vi "2014 Ball Detection.vi"(0 "Image In":T1) -> (1 "Annotated Image":T1, 2 "Ranked Objects":T3(array[cluster]) {"Score" format="%#.1g"})   [LabVIEW 2013]
uses:
  <vilib>/vision/Image Controls.llb/IMAQ Image.ctl
panel:
  in  "Std Devs":cluster{"Hue":dbl, "Sat":dbl, "Val":dbl}={"Hue"=4.0, "Sat"=6.0, "Val"=4.0}
  in  "Targets":i32=3
  in  "Area Size Limit %":dbl=0.4 format="%#_13g"
  out "loop time ms":u32=3805
  in  "Score Cutoff":dbl(slide)=70.58823529411765 scale=0.0..100.0
  in  "Color Components":T2={"Hue"={243.23333311080933, 20.233333110809326}, "Sat"={125.60287475585938, 242.93045043945312}, "Val"={83.88507843017578, 225.38158416748047}} {"Val" scale=0.0..255.0; "Sat" scale=0.0..255.0; "Hue" scale=0.0..255.0 scale format="%#_3g"}
  in  "Tabbed Info":enum32{"Debugging", "Details"}(tab)
  in  "Annotations":enum16{"None", "Good", "All"}(ring)=enum."Good"
  out "Initial Mask":T1(plugin-control)
  out "Fitted Mask":T1(plugin-control)
  out "Image":T1(plugin-control)
  # "Ranking Colors:\n1. green\n2. cyan\n3. magenta\n4. orange"
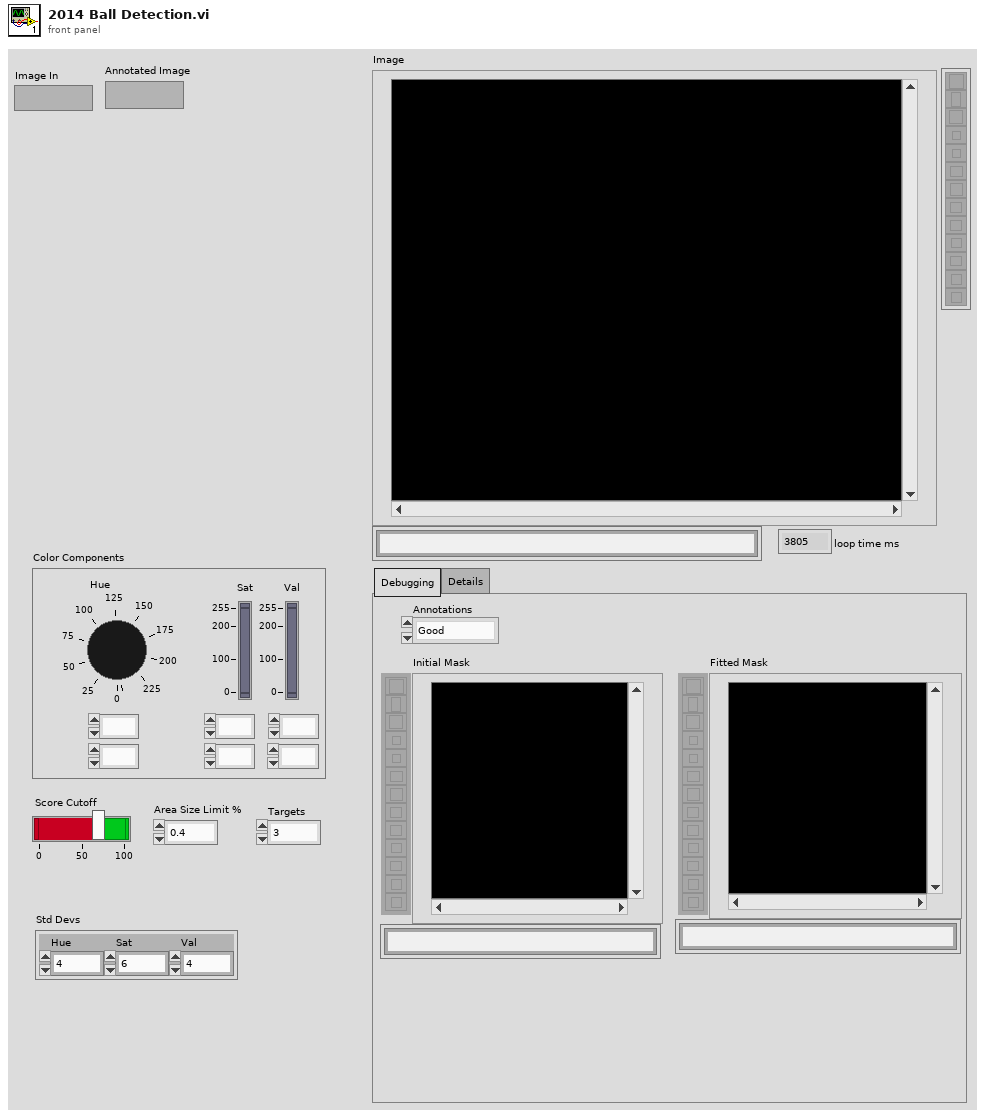
[diagram p1: front panel]
types:
  T1 = typedef "IMAQ Image.ctl" = refnum<image>
  T2 = cluster{"Hue":cluster{dbl, dbl}, "Sat":cluster{dbl, dbl}, "Val":cluster{dbl, dbl}}
  T3 = cluster{"Score":sgl, "Fitted Circle":cluster{"Center":cluster{"X":sgl, "Y":sgl}, "Radius":dbl, "Circle Rect":cluster{"L":sgl, "T":sgl, "R":sgl, "B":sgl}, "Roundness":dbl, "SNR (dB)":dbl}, "Search Rect":cluster{"L":sgl, "T":sgl, "R":sgl, "B":sgl}, "Details":cluster{"Edge":sgl, "Area":sgl, "Circ":sgl, "Diam":sgl}}[]
  T4 = cluster{cluster{dbl, dbl}, cluster{dbl, dbl}, cluster{dbl, dbl}}
  T5 = cluster{"Circle Found":bool, "Fitted Circle":cluster{"Center":cluster{"X":sgl, "Y":sgl}, "Radius":dbl, "Center":cluster{"X":sgl, "Y":sgl}, "Radius":dbl, "Roundness":dbl, "Strength":dbl, "SNR (dB)":dbl}, "Array":dbl[], "Sorted Data":dbl[][]}[]
  T6 = cluster{"Score":dbl, "Fitted Circle":cluster{"Center (Pixels)":cluster{"X":sgl, "Y":sgl}, "Radius (Pixels)":dbl, "Circle Rect":cluster{"Left":sgl, "Top":sgl, "Right":sgl, "Bottom":sgl}, "Roundness (RW)":dbl, "Average SNR (dB)":dbl}, "Search Rect":cluster{"Left":sgl, "Top":sgl, "Right":sgl, "Bottom":sgl}, "Details":cluster{"Edges":sgl, "Circ/Rect":sgl, "Diam/Diam":sgl, "Circularity":sgl}}[]
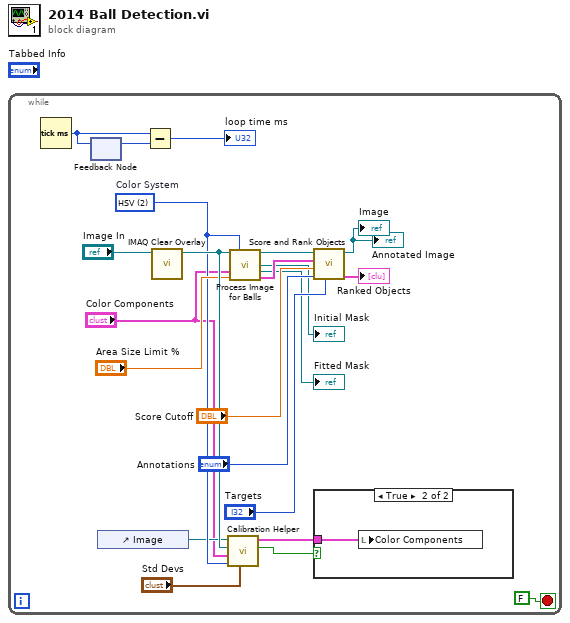
[diagram p0: block diagram]
diagram:
  n1 = while {
    stop <- FALSE stop-if-true
    w7 = u16 2 items=["RGB", "HSL", "HSV", "HSI"]  # Color System
    n2 = Tick Count (ms)() -> (millisecond timer value=w21:u32)
    n3 = feedback #1() -> (w20:u32)  [unwired: 1 in]
    n4 = feedback-in #1(w21) -> ()
    n5 = control-ref of="Image"() -> (w6:refnum<vi>)
    n6 = Subtract(x=w21, y=w20) -> (x-y=→"loop time ms":u32)
    n7 = call "IMAQ Clear Overlay"("Image"="Image In") -> ("Image Out"=w14:T1)  [unwired: 9 in, 1 out]
    n8 = call "Calibration Helper.vi"("Std Devs"="Std Devs", "Color Mode"=w7, "Color Components"="Color Components", "Image"=w14, "Image Ctl Refnum"=w6) -> ("Changed"=w3:bool, "output color"=w5:T4)  [unwired: 5 in]
    n9 = call "Process Image for Balls.vi"("Src Image"=w14, "Color Mode 2"=w7, "Color"="Color Components", "Area Cutoff %"="Area Size Limit %") -> ("Src Image Out"=w12:T1, "First Threshold"=→"Initial Mask":T1, "Fitted"=→"Fitted Mask":T1, "Potential"=w11:T5)  [unwired: 8 in]
    n10 = call "Score and Rank Objects.vi"("Targets"="Targets", "Annotations"="Annotations", "Score Limit"="Score Cutoff", "Object Info"=w11, "Image in"=w12) -> ("Object Info"=→"Ranked Objects":T6, "Annotated Image"=→"Image" →"Annotated Image":T1)  [unwired: 5 in]
    n11 = case shown="True" w3 {
      tunnel: w5 -> [_ w23]
      frame False {
      }
      frame True {
        n12 = local write "Color Components"(w23) -> ()
      }
    }
  }
